vi "Auton Drive Straight Helper.vi"(6 "PID gains":T11, 9 "Gyro Angle":dbl, 10 "Power":dbl, 11 "RobotDriveDevRef":T1) -> (1 "PID Out":dbl(graph), 2 "Motor Outputs":cluster{"Gyro Angle":dbl, "Gyro Angle":dbl}(graph), 3 "Set and Angle":cluster{"Gyro Angle":dbl, "Gyro Angle":dbl}(graph))   [LabVIEW 2014]
uses:
  <vilib>/Rock Robotics/WPI/RobotDrive/WPI_RobotDriveDevRef.ctl
  <vilib>/Rock Robotics/WPI/MotorControl/WPI_MotorControlDeviceRef.ctl
  <vilib>/Rock Robotics/WPI/MotorControl/WPI_MotorControlType.ctl
  <vilib>/Rock Robotics/SystemInterfaces/Typedef/FPGA_TypedefDigitalModule.ctl
  <vilib>/Rock Robotics/SystemInterfaces/DIO/FPGA_DIOPWMChannel.ctl
  <vilib>/Rock Robotics/WPI/PWM/WPI_PWMDeadband.ctl
  <vilib>/Rock Robotics/WPI/CAN/Jaguar/SubVIs/WPI_CANJaguar_ControlMode.ctl
  <vilib>/Rock Robotics/WPI/CAN/TalonSRX/WPI_CANTalonSRX_APIControlMode.ctl
  <vilib>/Rock Robotics/WPI/PWM/WPI_PWMTransform_ConPane.ctl
  GyroGlobal.vi
  <vilib>/addons/control/pid/pid.llb/PID (DBL).vi
  <vilib>/Rock Robotics/WPI/RobotDrive/WPI_RobotDriveArcadeDrive_Standard(NoSaturation).vi
  <vilib>/addons/control/pid/NI_PID_pid.lvlib
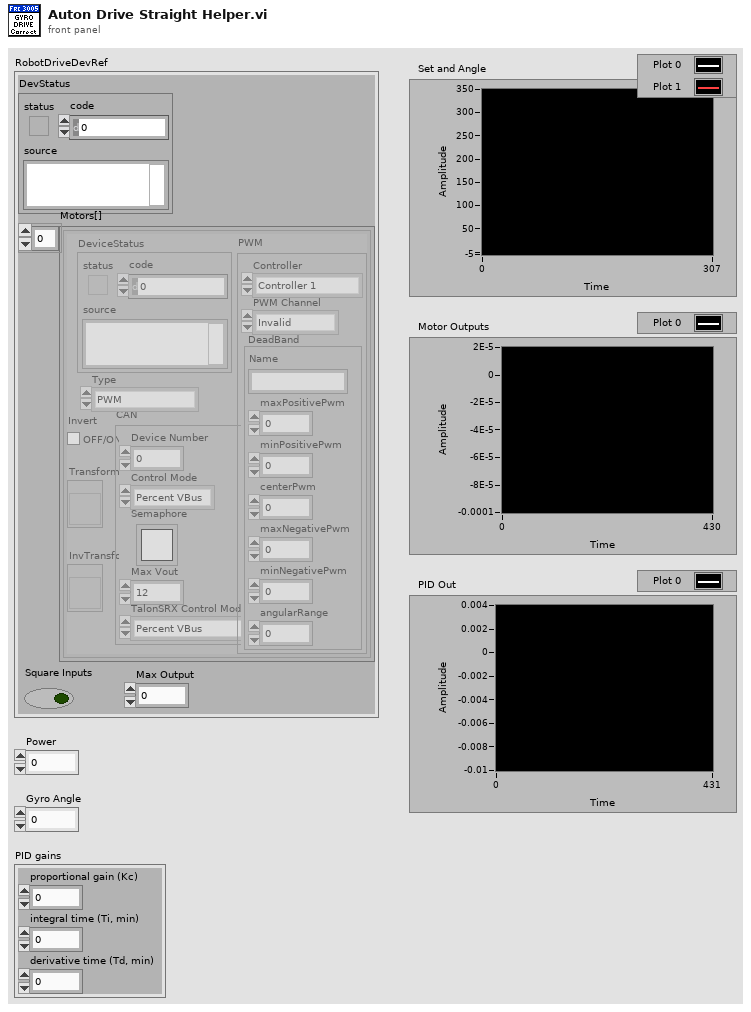
[diagram p1: front panel]
types:
  T1 = typedef "WPI_RobotDriveDevRef.ctl" = cluster{"DevStatus":errorcluster, "Motors[]":T2[], "Square Inputs":bool, "Max Output":dbl}
  T2 = typedef "WPI_MotorControlDeviceRef.ctl" = cluster{"DeviceStatus":errorcluster, "Type":T3, "PWM":cluster{"Controller":T4, "PWM Channel":T5, "DeadBand":T6}, "CAN":cluster{"Device Number":u8, "Control Mode":T7, "Semaphore":T8, "Max Vout":dbl, "TalonSRX Control Mode":T9}, "Invert":bool, "TransformRef":T10, "InvTransformRef":T10}
  T3 = typedef "WPI_MotorControlType.ctl" = enum16{"PWM", "CAN", "CANTalonSRX"}
  T4 = typedef "FPGA_TypedefDigitalModule.ctl" = enum16{"Controller 1"}
  T5 = typedef "FPGA_DIOPWMChannel.ctl" = enum8{"PWM 0", "PWM 1", "PWM 2", "PWM 3", "PWM 4", "PWM 5", "PWM 6", "PWM 7", "PWM 8", "PWM 9", "PWM MXP 0", "PWM MXP 1", "PWM MXP 2", "PWM MXP 3", "PWM MXP 4", "PWM MXP 5", "PWM MXP 6", "PWM MXP 7", "PWM MXP 8", "PWM MXP 9", "Invalid"}
  T6 = typedef "WPI_PWMDeadband.ctl" = cluster{"Name":string, "maxPositivePwm":i32, "minPositivePwm":i32, "centerPwm":i32, "maxNegativePwm":i32, "minNegativePwm":i32, "angularRange":u16}
  T7 = typedef "WPI_CANJaguar_ControlMode.ctl" = enum8{"Percent VBus", "Current", "Speed", "Position", "Voltage"}
  T8 = typedef "Semaphore RefNum" = refnum<k1>
  T9 = typedef "WPI_CANTalonSRX_APIControlMode.ctl" = enum8{"Percent VBus", "Speed", "Position", "Slave", "Unchanged / Invalid"}
  T10 = typedef "WPI_PWMTransform_ConPane.ctl" = refnum<vi>
  T11 = cluster{"proportional gain (Kc)":dbl, "integral time (Ti, min)":dbl, "derivative time (Td, min)":dbl}
  T12 = cluster{"Motor Values[0]":dbl, "Motor Values[1]":dbl}
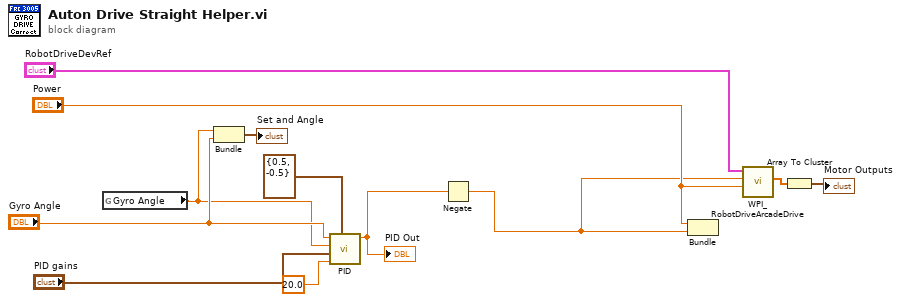
[diagram p0: block diagram]
diagram:
  n1 = global read "GyroGlobal.vi" "Gyro Angle"() -> (w10:dbl)
  n2 = Bundle("Gyro Angle"=w10, "Gyro Angle"="Gyro Angle") -> (→"Set and Angle":cluster{"Gyro Angle":dbl, "Gyro Angle":dbl})  [unwired: 1 in]
  n3 = call-poly <vilib>:"PID.vi"("output range"=cluster{"output high":dbl, "output low":dbl} {"output high"=0.5, "output low"=-0.5}, "dt (s)"=20.0, "PID gains"="PID gains", "process variable"=w10, "setpoint"="Gyro Angle") -> ("output"=w5:dbl)  [unwired: 5 in, 1 out]
  "PID Out" <- w5
  n4 = Negate(x=w5) -> (-x=w1:dbl)
  n5 = Bundle("Power"="Power", w1) -> ()  [unwired: 1 in, 1 out]
  n6 = call-poly <vilib>:"WPI_RobotDriveArcadeDrive.vi"("Y axis value"="Power", "X axis value"=w1, "RobotDriveDevRef"="RobotDriveDevRef") -> ("Motor Values"=w3:dbl[])  [unwired: 6 in, 2 out]
  n7 = Array To Cluster(array=w3) -> (cluster=→"Motor Outputs":T12)
